vi "Build Frequency List.vi"(0 "start":dbl format="%#_13g", 5 "step":dbl format="%#_13g", 9 "stop":dbl format="%#_13g", 11 "error in (no error)":errorcluster) -> (4 "Frequency List":dbl[](array[numeric]), 15 "error out":errorcluster)   [LabVIEW 2023, in "RFCalAndFixtureCharact.Common.lvlib"]
uses:
  RFCalAndFixtureCharact.Common.lvlib
  <vilib>/Analysis/1siggen.llb/Ramp Pattern by Delta.vi
  <vilib>/Analysis/NI_AALBase.lvlib
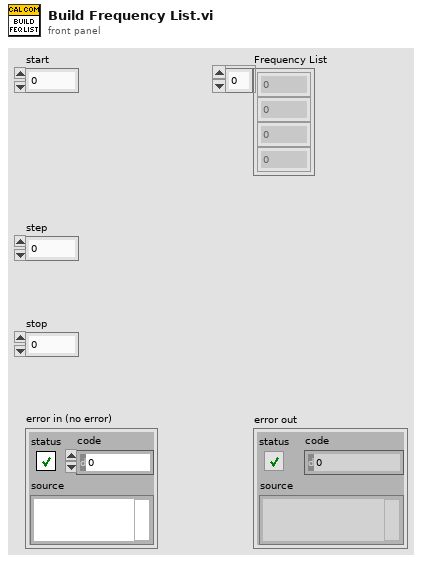
[diagram p1: front panel]
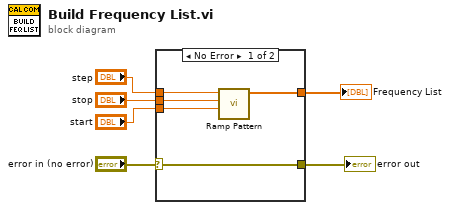
[diagram p0: block diagram]
diagram:
  n1 = case shown="No Error" "error in (no error)" {
    selector: "error in (no error)" -> [w11 w12]
    tunnel: [w11 w12] -> w5
    tunnel: "start" -> [w9 _]
    tunnel: "stop" -> [w8 _]
    tunnel: "step" -> [w10 _]
    tunnel: [w7 _] -> w1
    frame No Error {
      n2 = call-poly <vilib>:"Ramp Pattern.vi"("start"=w9, "end"=w8, "delta"=w10) -> ("Ramp Pattern"=w7:dbl[])  [unwired: 6 in, 2 out]
    }
    frame Error {
    }
  }
  "error out" <- w5
  "Frequency List" <- w1
